vi "Condition Name Msg.vi"(4 "Name":string, 6 "Terminals (All Msg Output)":T2, 8 "error in":errorcluster, 9 "Terminals (All Msg Input)":T2, 10 "Name Msg":T1) -> (0 "error out":errorcluster)   [LabVIEW 2020, in "_Rescript.lvlib" / "Msg.lvlib" / "Msg.lvclass"]
uses:
  Msg.lvclass
  Terminals.ctl
  Name Msg.ctl
  <vilib>/Utility/traverseref.llb/TRef TravTarget.ctl
  _Rescript.lvlib
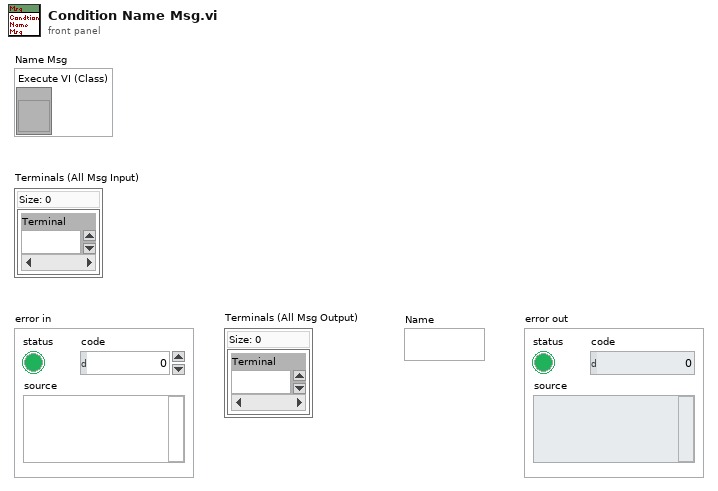
[diagram p1: front panel]
types:
  T1 = typedef "_Rescript.lvlib/Msg.lvlib/Msg.lvclass/Name Msg.ctl" = cluster{"Execute VI (Class)":refnum<vi>}
  T2 = typedef "_Rescript.lvlib/Terminals.ctl" = set{i32}
  T3 = typedef "TRef TravTarget.ctl" = enum16{"FP", "BD", "Other"}
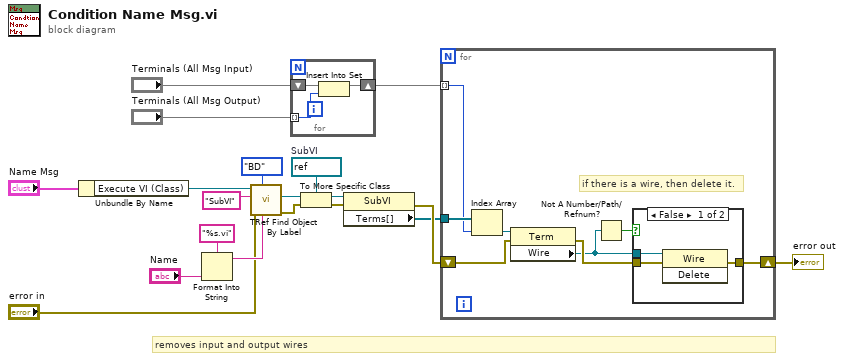
[diagram p0: block diagram]
diagram:
  w18 = refnum<vi> refnum  # SubVI
  # "removes input and output wires"
  n1 = Unbundle By Name("Name Msg") -> ("Execute VI (Class)"=w2:refnum<vi>)
  n2 = Format Into String(format string="%s.vi", "Name") -> (resulting string=w9:string)  [unwired: 2 in, 1 out]
  n3 = call <vilib>:"TRef Find Object By Label.vi"("Label"=w9, "Traverse Target"=TRef_TravTarget."BD", "error in (no error)"="error in", "Class Name"="SubVI", "VI Ref"=w2) -> ("error out"=w17:errorcluster, "Found Obj Ref"=w11:refnum<vi>)  [unwired: 3 in, 2 out]
  n4 = for {
    shift-right: [w21] -> w1
    shift-left: "Terminals (All Msg Input)" -> [w22]
    tunnel: "Terminals (All Msg Output)" -> [w20] mode=indexing
    n5 = Insert Into Set(10:w20, 11:w22) -> (3:w21:T2)  [unwired: 1 out]
  }
  n6 = To More Specific Class(target class=w18, reference=w11, error in=w17) -> (specific class reference=w15:refnum<vi>, error out=w14:errorcluster)
  n7 = property class="SubVI"(reference=w15, error in=w14) -> (error out=w13:errorcluster, "Terms[]"=w8:refnum<vi>[])  [unwired: 1 out]
  n8 = for {
    tunnel: w8 -> [w30]
    tunnel: w1 -> [w29] mode=indexing
    shift-right: [w28] -> w7
    shift-left: w13 -> [w26]
    # "if there is a wire, then delete it."
    n9 = Index Array(array=w30, index=w29) -> (element=w27:refnum<vi>)
    n10 = property class="Term"(reference=w27, error in=w26) -> (error out=w25:errorcluster, "Wire"=w24:refnum<vi>)  [unwired: 1 out]
    n11 = Not A Number/Path/Refnum?(number/path/refnum=w24) -> (NaN/Path/Refnum?=w23:bool)
    n12 = case shown="False" w23 {
      tunnel: [w33 w34] -> w28
      tunnel: w24 -> [w32 _]
      tunnel: w25 -> [w31 w34]
      frame False {
        n13 = invoke class="Wire" method="Delete"(reference=w32, error in=w31) -> (error out=w33:errorcluster)  [unwired: 1 in, 2 out]
      }
      frame True {
      }
    }
  }
  "error out" <- w7
